vi "NMRvmeCard1.vi"() -> ()   [LabVIEW 2013]
uses:
  <vilib>/Utility/file.llb/Read From Spreadsheet File (DBL).vi
  <vilib>/Analysis/NI_AALBase.lvlib
panel:
  out "Telnet error out":errorcluster
  in  "Real/quad Q curve":bool=TRUE
  out "Temperature (C)":dbl(graph)=24.12
  out "+3V supply":dbl=3.245 format="%_4g"
  out "Temp (C)":dbl=24.12 format="%_4g"
  in  "RemovePed":bool=TRUE
  in  "IF / LOG Det":bool=TRUE
  in  "Q curve file":string="realback213.txt"
  out "File name 2":string="C:\\users\\plm\\Desktop\\rssmt\\realback213.txt"
  in  "AutoBaseline":bool
  out "RF OK":bool=TRUE
  out "Peak area (V-MHz)":sgl=0.0012676906 format="%.5f"
  in  "Gauss Fit":bool=TRUE
  out "NMR Graph + Fit":cluster{cluster{dbl, "Numeric":dbl}[]}[](graph)=[{[{224.37, "Numeric"=0.019981380952380993}, {224.372, "Numeric"=0.01883813333333495}, {224.374, "Numeric"=0.016386885714283997}, {224.376, "Numeric"=0.008227638095238155}, {224.37800000000001, "Numeric"=0.00466039047619202}, {224.38, "Numeric"=0.006385142857141357}, {224.382, "Numeric"=0.0035018952380952402}, {224.38400000000001, "Numeric"=0.005910647619049087}, {224.386, "Numeric"=0.004711399999998608}, {224.388, "Numeric"=0.005604152380952493}, {224.39000000000001, "Numeric"=0.0029889047619062}, {224.392, "Numeric"=0.006765657142855813}, {224.394, "Numeric"=0.00683440952380954}, {224.39600000000002, "Numeric"=0.006795161904763159}, {224.398, "Numeric"=0.002147914285713117}, {224.4, "Numeric"=0.002992666666666621}, {224.40200000000002, "Numeric"=-0.0024705809523797445}, {224.404, "Numeric"=0.00015817142857038526}, {224.406, "Numeric"=0.0007789238095238871}, {224.40800000000002, "Numeric"=-0.0025083238095228557}, {224.41, "Numeric"=-0.012503571428572361}, {224.412, "Numeric"=-0.009706819047619015}, {224.41400000000002, "Numeric"=-0.018818066666665807}, {224.416, "Numeric"=-0.01873731428571512}, {224.418, "Numeric"=-0.019264561904761987}, {224.42000000000002, "Numeric"=-0.012999809523808725}, {224.422, "Numeric"=-0.009943057142857946}, {224.424, "Numeric"=-0.00489430476190479}, {224.426, "Numeric"=-0.00615355238095111}, {224.428, "Numeric"=-0.0050208000000006485}, {224.43, "Numeric"=0.006503952380952323}, {224.432, "Numeric"=-0.003579295238094162}, {224.434, "Numeric"=-0.0057705428571434726}, {224.436, "Numeric"=-0.008969790476190571}, {224.438, "Numeric"=-0.009677038095237117}, {224.44, "Numeric"=-0.005792285714286235}, {224.442, "Numeric"=-0.004715533333333498}, {224.444, "Numeric"=-0.016146780952380223}, {224.446, "Numeric"=-0.01998602857142907}, {224.448, "Numeric"=-0.013633276190476386}, {224.45, "Numeric"=-0.009988523809523243}, {224.452, "Numeric"=0.002948228571428255}, {224.454, "Numeric"=0.009376980952380683}, {224.456, "Numeric"=0.013697733333333725}, {224.458, "Numeric"=0.01901048571428548}, {224.46, "Numeric"=0.030415238095237777}, {224.462, "Numeric"=0.037711990476190685}, {224.464, "Numeric"=0.0454007428571426}, {224.466, "Numeric"=0.060881495238094864}, {224.468, "Numeric"=0.07065424761904769}, {224.47, "Numeric"=0.07911899999999972}, {224.472, "Numeric"=0.07487575238095191}, {224.474, "Numeric"=0.06432450476190474}, {224.476, "Numeric"=0.055565257142856955}, {224.478, "Numeric"=0.03969800952380907}, {224.48, "Numeric"=0.019822761904761673}, {224.482, "Numeric"=0.012039514285714098}, {224.484, "Numeric"=0.0025482666666661463}, {224.486, "Numeric"=-0.004650980952381451}, {224.488, "Numeric"=-0.008758228571428682}, {224.49, "Numeric"=-0.009773476190476815}, {224.492, "Numeric"=-0.0021967238095244018}, {224.494, "Numeric"=-0.001127971428571451}, {224.496, "Numeric"=-0.0037672190476198773}, {224.498, "Numeric"=-0.0021144666666660606}, {224.5, "Numeric"=0.00043028571428570164}, {224.502, "Numeric"=-0.0007329619047626916}, {224.504, "Numeric"=0.0017957904761913349}, {224.506, "Numeric"=0.004616542857142707}, {224.508, "Numeric"=-0.00017070476190575782}, {224.51, "Numeric"=-0.001065952380951492}, {224.512, "Numeric"=-0.0026691999999999922}, {224.514, "Numeric"=-0.00778044761904867}, {224.516, "Numeric"=-0.0050996952380941585}, {224.518, "Numeric"=-0.005226942857142848}, {224.51999999999998, "Numeric"=-0.002862190476190984}, {224.522, "Numeric"=-0.004705438095236949}, {224.524, "Numeric"=-0.004856685714285773}, {224.52599999999998, "Numeric"=0.0025840666666660603}, {224.528, "Numeric"=0.009216819047620357}, {224.53, "Numeric"=0.0054415714285713495}, {224.53199999999998, "Numeric"=0.0009583238095230262}, {224.534, "Numeric"=-0.00043292380952248636}, {224.536, "Numeric"=0.0008678285714284759}, {224.53799999999998, "Numeric"=0.004360580952380025}, {224.54, "Numeric"=0.005645333333334857}, {224.542, "Numeric"=0.008922085714285575}, {224.54399999999998, "Numeric"=0.004790838095237049}, {224.546, "Numeric"=0.00255159047619202}, {224.548, "Numeric"=-0.009795657142857232}, {224.54999999999998, "Numeric"=-0.005650904761906031}, {224.552, "Numeric"=-0.0035141523809506803}, {224.554, "Numeric"=-0.004185400000000136}, {224.55599999999998, "Numeric"=-0.009264647619048945}, {224.558, "Numeric"=-0.0021518952380935015}, {224.56, "Numeric"=0.004852857142857059}, {224.56199999999998, "Numeric"=0.005449609523808043}, {224.564, "Numeric"=0.002138361904763719}, {224.566, "Numeric"=0.003119114285714139}, {224.56799999999998, "Numeric"=0.003891866666664966}, {224.57, "Numeric"=0.0027566190476209307}]}, {[{224.37, "Numeric"=4.996479157121043e-53}, {224.372, "Numeric"=5.331405671308769e-51}, {224.374, "Numeric"=5.17637625627724e-49}, {224.376, "Numeric"=4.573160046621097e-47}, {224.37800000000001, "Numeric"=3.6763209752488545e-45}, {224.38, "Numeric"=2.6891615986254814e-43}, {224.382, "Numeric"=1.7898920413809642e-41}, {224.38400000000001, "Numeric"=1.0840348153164538e-39}, {224.386, "Numeric"=5.974011869109323e-38}, {224.388, "Numeric"=2.9956797876429715e-36}, {224.39000000000001, "Numeric"=1.3668824093475549e-34}, {224.392, "Numeric"=5.675098152549435e-33}, {224.394, "Numeric"=2.143986553114384e-31}, {224.39600000000002, "Numeric"=7.370164723645891e-30}, {224.398, "Numeric"=2.3053601888071056e-28}, {224.4, "Numeric"=6.561556019740437e-27}, {224.40200000000002, "Numeric"=1.6993441869680083e-25}, {224.404, "Numeric"=4.004629265065266e-24}, {224.406, "Numeric"=8.587163671653244e-23}, {224.40800000000002, "Numeric"=1.6754968737140568e-21}, {224.41, "Numeric"=2.97470538953919e-20}, {224.412, "Numeric"=4.805634713914891e-19}, {224.41400000000002, "Numeric"=7.064216637569256e-18}, {224.416, "Numeric"=9.44895367190872e-17}, {224.418, "Numeric"=1.1500319007026123e-15}, {224.42000000000002, "Numeric"=1.2736277485103554e-14}, {224.422, "Numeric"=1.2834578034111644e-13}, {224.424, "Numeric"=1.1768663207807158e-12}, {224.426, "Numeric"=9.819268406815462e-12}, {224.428, "Numeric"=7.45482728048275e-11}, {224.43, "Numeric"=5.149943891555167e-10}, {224.432, "Numeric"=3.2372323103657745e-09}, {224.434, "Numeric"=1.851619273182036e-08}, {224.436, "Numeric"=9.636869461784531e-08}, {224.438, "Numeric"=4.5638011879864213e-07}, {224.44, "Numeric"=1.966635685025587e-06}, {224.442, "Numeric"=7.711299494825998e-06}, {224.444, "Numeric"=2.7512983238559256e-05}, {224.446, "Numeric"=8.932113926203351e-05}, {224.448, "Numeric"=0.0002638622619953867}, {224.45, "Numeric"=0.0007092621201427087}, {224.452, "Numeric"=0.0017347732149989375}, {224.454, "Numeric"=0.0038608693662806003}, {224.456, "Numeric"=0.007818689455772231}, {224.458, "Numeric"=0.014407521558145594}, {224.46, "Numeric"=0.024157447780126944}, {224.462, "Numeric"=0.03685694020534238}, {224.464, "Numeric"=0.05116747240443425}, {224.466, "Numeric"=0.06463609450757957}, {224.468, "Numeric"=0.0742955338825832}, {224.47, "Numeric"=0.07770639578127585}, {224.472, "Numeric"=0.0739532527937006}, {224.474, "Numeric"=0.0640419066890079}, {224.476, "Numeric"=0.050463536567084744}, {224.478, "Numeric"=0.036182416660317206}, {224.48, "Numeric"=0.02360608219203614}, {224.482, "Numeric"=0.014013825865809171}, {224.484, "Numeric"=0.007570001678288115}, {224.486, "Numeric"=0.0037208459705686692}, {224.488, "Numeric"=0.0016641553514492678}, {224.49, "Numeric"=0.0006772554318493228}, {224.492, "Numeric"=0.0002507942558558377}, {224.494, "Numeric"=8.450630852905024e-05}, {224.496, "Numeric"=2.59099833493484e-05}, {224.498, "Numeric"=7.228556737491606e-06}, {224.5, "Numeric"=1.8350272242305546e-06}, {224.502, "Numeric"=4.2387703390211724e-07}, {224.504, "Numeric"=8.90930278726135e-08}, {224.506, "Numeric"=1.7039388635256535e-08}, {224.508, "Numeric"=2.965314459410487e-09}, {224.51, "Numeric"=4.69563098204409e-10}, {224.512, "Numeric"=6.765869563309472e-11}, {224.514, "Numeric"=8.870737740659163e-12}, {224.516, "Numeric"=1.0582842087595977e-12}, {224.518, "Numeric"=1.1488183111935901e-13}, {224.51999999999998, "Numeric"=1.1347673718942467e-14}, {224.522, "Numeric"=1.0199262936518405e-15}, {224.524, "Numeric"=8.341366305650706e-17}, {224.52599999999998, "Numeric"=6.20743321960535e-18}, {224.528, "Numeric"=4.2033289216604396e-19}, {224.53, "Numeric"=2.5898890134957684e-20}, {224.53199999999998, "Numeric"=1.4520293268026514e-21}, {224.534, "Numeric"=7.407575384802874e-23}, {224.536, "Numeric"=3.4386124328008906e-24}, {224.53799999999998, "Numeric"=1.4524354344352625e-25}, {224.54, "Numeric"=5.582347908555169e-27}, {224.542, "Numeric"=1.9522859135246242e-28}, {224.54399999999998, "Numeric"=6.2126430133960394e-30}, {224.546, "Numeric"=1.7989365057346025e-31}, {224.548, "Numeric"=4.7398186788252815e-33}, {224.54999999999998, "Numeric"=1.1363551343839747e-34}, {224.552, "Numeric"=2.478979219883001e-36}, {224.554, "Numeric"=4.920827616420029e-38}, {224.55599999999998, "Numeric"=8.888119269018469e-40}, {224.558, "Numeric"=1.4607908954776238e-41}, {224.56, "Numeric"=2.1846038284560563e-43}, {224.56199999999998, "Numeric"=2.9727869424363234e-45}, {224.564, "Numeric"=3.6809620192977223e-47}, {224.566, "Numeric"=4.147298983609085e-49}, {224.56799999999998, "Numeric"=4.2518292134929295e-51}, {224.57, "Numeric"=3.966365529511812e-53}]}]
  in  "Amp of Q curve":dbl=0.9999999999999999 min=0.0 max=7.0 step=0.01 format="%_3f"
  in  "Subtract Q curve":bool=TRUE
  in  "Adjust Tune":bool
  out "Pedestal Offset":dbl(graph)=0.7186800000000002
  out "Pedestal Difference":dbl(graph)=0.003027333333333382
  out "# Good Spectra":i32=97
  in  "Quality cuts":bool=TRUE
  out "Pedestal OK":bool=TRUE
  out "Sweep #":i32=127
  out "1st Sweep":bool
  out "ADC volts OK":bool=TRUE
  out "Peak Height Distribution":cluster{"Y":dbl[], "Y":dbl[]}[](graph)=[{"Y"=[0.04386130127363737, 0.04436487009623908, 0.0448684389188408, 0.04537200774144251, 0.04587557656404422, 0.04637914538664594, 0.04688271420924765, 0.04738628303184937, 0.04788985185445108, 0.048393420677052795, 0.048896989499654514, 0.049400558322256226, 0.049904127144857945, 0.050407695967459656, 0.050911264790061375, 0.05141483361266309, 0.0519184024352648, 0.05242197125786652, 0.05292554008046823, 0.05342910890306995, 0.05393267772567166, 0.05443624654827338, 0.05493981537087509, 0.0554433841934768, 0.05594695301607852, 0.05645052183868023, 0.05695409066128195, 0.057457659483883664, 0.057961228306485375, 0.058464797129087094, 0.058968365951688806, 0.059471934774290525, 0.059975503596892236, 0.060479072419493955, 0.06098264124209567, 0.06148621006469738, 0.0619897788872991, 0.06249334770990081, 0.06299691653250253, 0.06350048535510425, 0.06400405417770595, 0.06450762300030767, 0.06501119182290939, 0.0655147606455111, 0.06601832946811281, 0.06652189829071453, 0.06702546711331625, 0.06752903593591796, 0.06803260475851967, 0.06853617358112139, 0.0690397424037231, 0.06954331122632482, 0.07004688004892654, 0.07055044887152824, 0.07105401769412996, 0.07155758651673168, 0.0720611553393334, 0.0725647241619351, 0.07306829298453682, 0.07357186180713854, 0.07407543062974024, 0.07457899945234196, 0.07508256827494368, 0.0755861370975454, 0.0760897059201471, 0.07659327474274882, 0.07709684356535054, 0.07760041238795225, 0.07810398121055397, 0.07860755003315568, 0.0791111188557574, 0.07961468767835911, 0.08011825650096083, 0.08062182532356255, 0.08112539414616425, 0.08162896296876597, 0.08213253179136769, 0.08263610061396941, 0.08313966943657111, 0.08364323825917283, 0.08414680708177455, 0.08465037590437625, 0.08515394472697797, 0.08565751354957969, 0.0861610823721814, 0.08666465119478312, 0.08716822001738483, 0.08767178883998655, 0.08817535766258826, 0.08867892648518998, 0.0891824953077917, 0.0896860641303934, 0.09018963295299512, 0.09069320177559684, 0.09119677059819856, 0.09170033942080026, 0.09220390824340198, 0.0927074770660037, 0.0932110458886054, 0.09371461471120712], "Y"=[1.0, 0.0, 0.0, 0.0, 0.0, 0.0, 2.0, 0.0, 0.0, 0.0, 0.0, 0.0, 0.0, 0.0, 0.0, 0.0, 0.0, 0.0, 0.0, 0.0, 0.0, 0.0, 2.0, 1.0, 0.0, 0.0, 0.0, 0.0, 1.0, 0.0, 0.0, 3.0, 0.0, 2.0, 0.0, 1.0, 0.0, 1.0, 1.0, 0.0, 0.0, 0.0, 2.0, 2.0, 1.0, 1.0, 1.0, 2.0, 1.0, 0.0, 6.0, 1.0, 1.0, 1.0, 2.0, 2.0, 5.0, 0.0, 3.0, 3.0, 4.0, 1.0, 2.0, 0.0, 3.0, 2.0, 1.0, 2.0, 3.0, 2.0, 0.0, 3.0, 1.0, 0.0, 0.0, 1.0, 2.0, 2.0, 1.0, 1.0, 1.0, 2.0, 0.0, 1.0, 1.0, 2.0, 0.0, 3.0, 1.0, 1.0, 0.0, 1.0, 0.0, 0.0, 2.0, 0.0, 0.0, 0.0, 1.0, 1.0]}]
  in  "# of Sweeps":i32=1000
  out "S/N":dbl=7.101836430067523 format="%_3g"
  out "Peak mean (V)":dbl=0.07363174247132291 format="%_4g"
  out "Peak Height":dbl(graph)=0.0777085900348737
  in  "Raw Data":bool=TRUE
  in  "Tank RF":bool=TRUE
  in  "IF Atten (dB)":i8=9 min=0 max=31 step=1
  in  "IFoffset (V)":dbl=6.713 min=-0.0 max=8.0 step=0.001 format="%.4f"
  in  "Tune  (V)":dbl=2.6299999999999994 min=0.0 max=5.0 step=0.001 format="%.4f"
  in  "Hi / Lo IF Gain":bool
  out "Voltage Array":sgl[](array[numeric])=[0.7467, 0.7452, 0.7424, 0.7339, 0.73, 0.7314, 0.7282, 0.7303, 0.7288, 0.7294, 0.7265, 0.73, 0.7298, 0.7295, 0.7246, 0.7252, 0.7195, 0.7219, 0.7223, 0.7188, 0.7086, 0.7112, 0.7019, 0.7018, 0.7011, 0.7072, 0.7101, 0.715, 0.7136, 0.7146, 0.726, 0.7158, 0.7135, 0.7102, 0.7094, 0.7132, 0.7142, 0.7027, 0.6988, 0.7051, 0.7087, 0.7216, 0.728, 0.7323, 0.7376, 0.749, 0.7563, 0.764, 0.7795, 0.7893, 0.7978, 0.7936, 0.7831, 0.7744, 0.7586, 0.7388, 0.7311, 0.7217, 0.7146, 0.7106, 0.7097, 0.7174, 0.7186, 0.7161, 0.7179, 0.7206, 0.7196, 0.7223, 0.7253, 0.7207, 0.72, 0.7186, 0.7137, 0.7166, 0.7167, 0.7193, 0.7177, 0.7178, 0.7255, 0.7324, 0.7289, 0.7247, 0.7236, 0.7252, 0.729, 0.7306, 0.7342, 0.7304, 0.7285, 0.7165, 0.721, 0.7235, 0.7232, 0.7185, 0.726, 0.7334, 0.7344, 0.7315, 0.7329, 0.7341, 0.7334] format="%.4f"
  in  "Invert Polarity":bool
  out "Pedestal Diff (V)":sgl=0.0030273334 format="%.3f"
  out "Peak amp (V)":sgl=0.07770859 format="%.3f"
  in  "Save Data to File":bool
  in  "RF Level (dBm)":dbl min=-10.0 max=10.0 step=0.1 format="%.2f"
  out "SMT error out":errorcluster
  out "Sample RMS (V)":dbl=0.001420792079207921 format="%.4f"
  in  "# Sample/step":i32=100 min=1 max=1000 step=100
  in  "Step Width (MHz)":dbl=0.002 min=0.0 max=1000.0 step=0.0005 format="%.4f"
  in  "Freq Span (MHz)":dbl=0.2 min=0.0 max=3000.0 step=0.1 format="%.3f"
  in  "Center Freq (MHz)":dbl=224.47 min=0.005 max=6000.0 step=0.1 format="%.3f"
  in  "Sweep Mode":u16(ring)=3 items=["Off", "Single", "Auto", "Step"]
  in  "GPIB Addr (28)":refnum<visa-resource-name>="GPIB0::28::INSTR"
  # "E1039 Prototype NMR Control Panel"
  # "Settings"
  # "D\nA\nC"
  # "R\nF\n\nG\nE\nN \n\n+\n\nI\nF"
  # "A\nD\nC"
  # "D\nA\nT\nA\n\n+\n\nA \nN\nA\nL\nY\nS\nI\nS"
  # "I\n/\nO"
  # "Results"
  # "A\nv\ne\nr\na\ng\ne"
  # "S\nw\ne\ne\np"
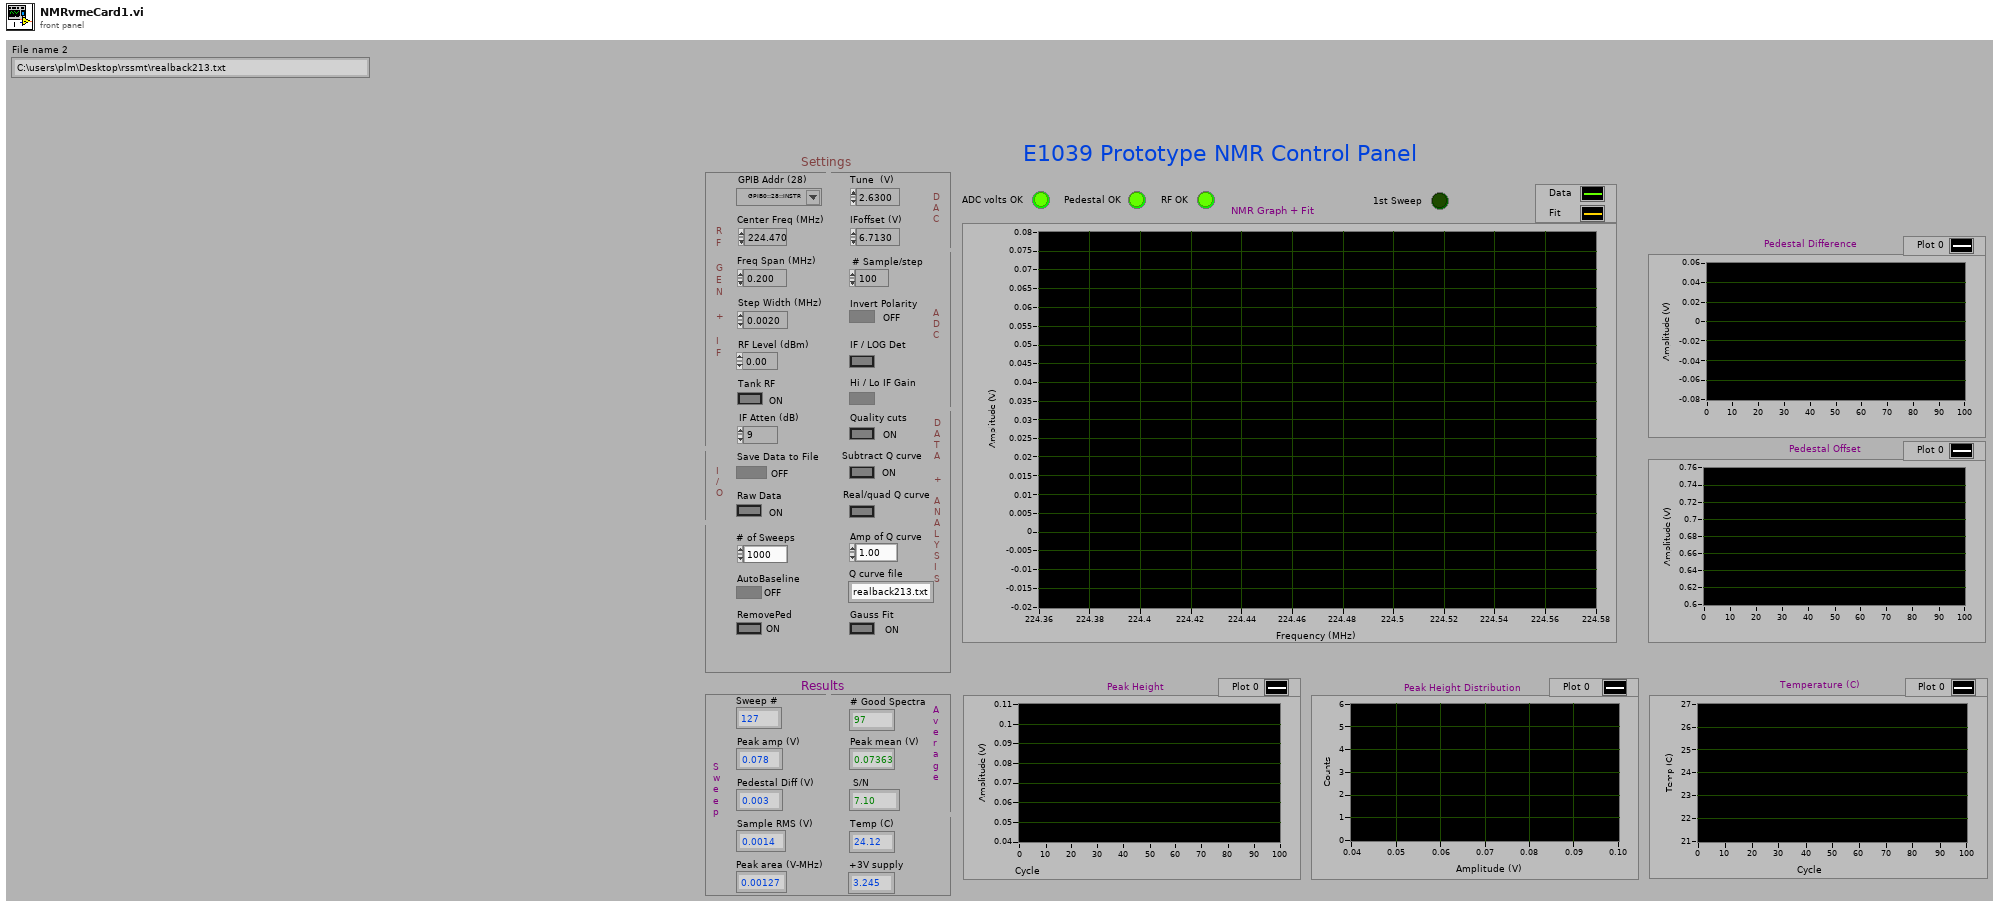
[diagram p1: front panel]
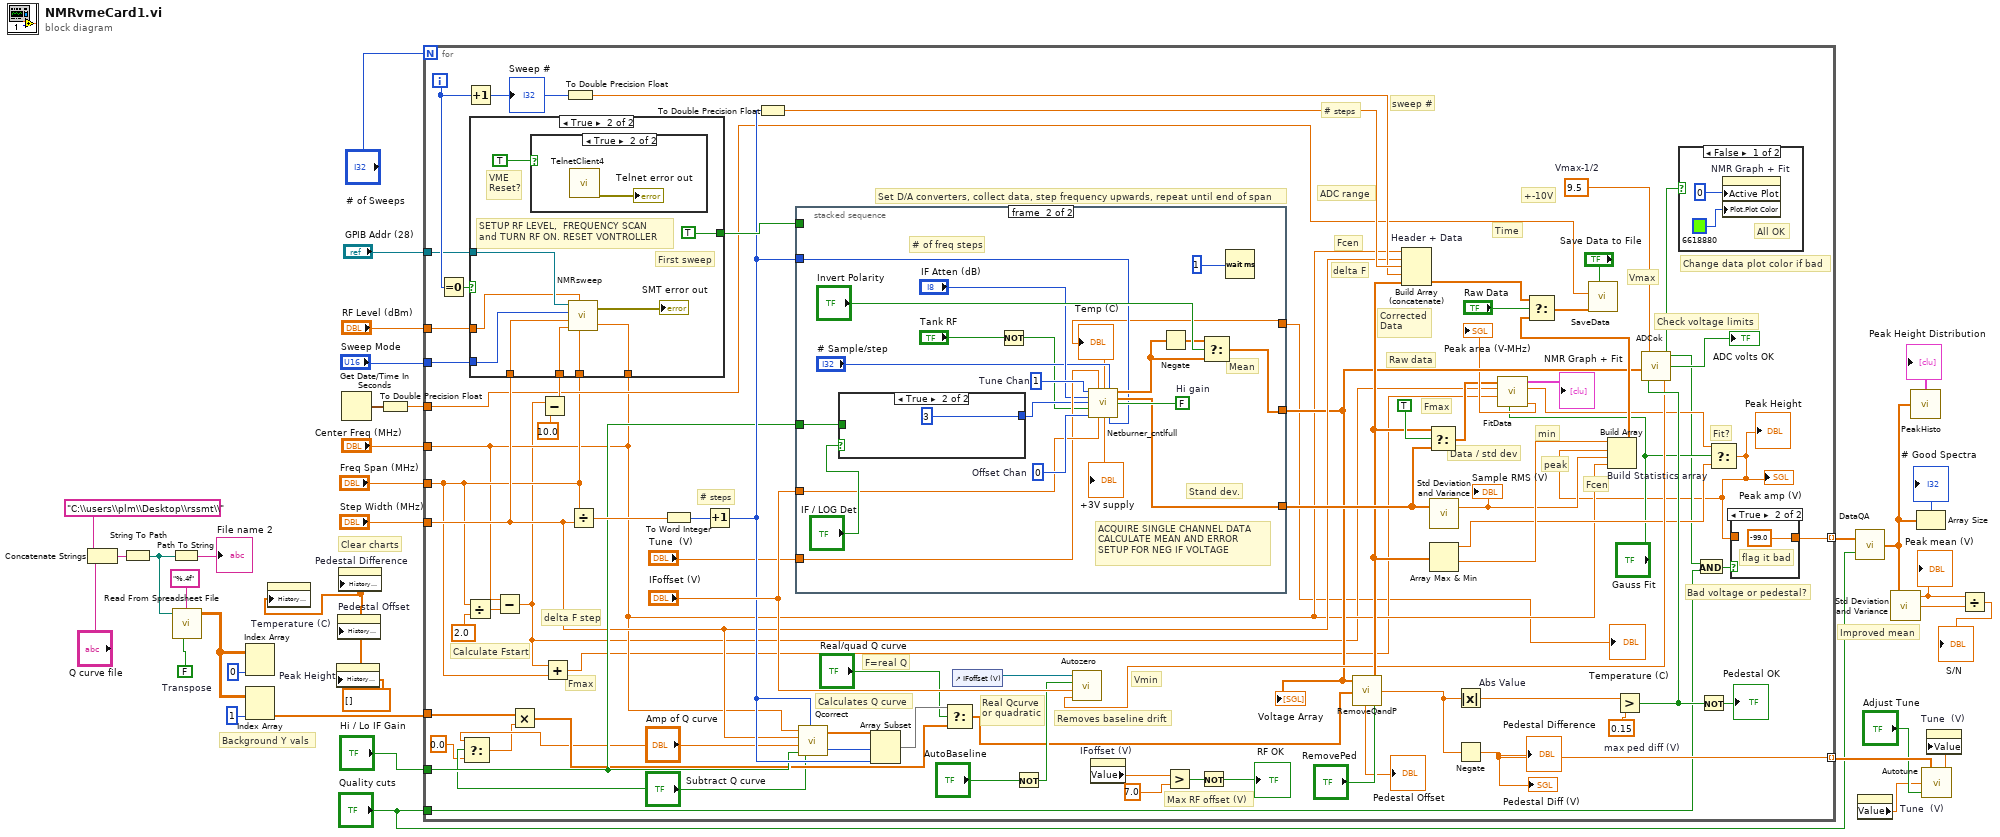
[diagram p0: block diagram]
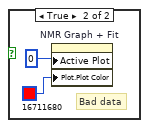
[diagram p2: hidden frame]
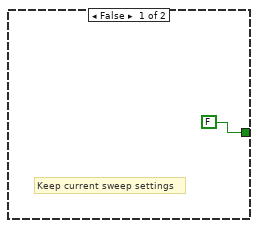
[diagram p4: hidden frame]
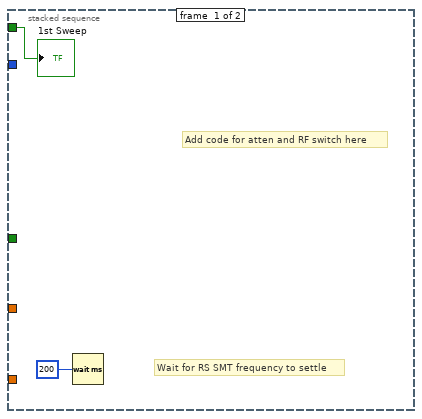
[diagram p6: hidden frame]
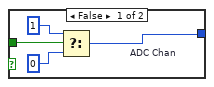
[diagram p7: hidden frame]
diagram:
  w12 = FALSE  # Transpose
  w4 = dbl[] []
  # "Background Y vals"
  # "Clear charts"
  # "Improved mean"
  n1 = Concatenate Strings "Concatenate Strings"("C:\\users\\plm\\Desktop\\rssmt\\", "Q curve file") -> (w15:string)
  n2 = String To Path(string=w15) -> (path=w11:path)
  n3 = Path To String(path=w11) -> (string=→"File name 2":string)
  n4 = call-poly <vilib>:"Read From Spreadsheet File.vi"("transpose (no:F)"=w12, "format (%.3f)"="%.4f", "file path (dialog if empty)"=w11) -> ("all rows"=w10:dbl[][])  [unwired: 4 in, 4 out]
  n5 = Index Array "Index Array"(array=w10, index (col)=0) -> ()  [unwired: 1 in, 1 out]
  n6 = Index Array(array=w10, index (col)=1) -> (element=w5:dbl[])  [unwired: 1 in]
  n7 = property on="Temperature (C)" class="WFChart (strict)"("History Data"=w4) -> ()  [unwired: 2 in, 2 out]
  n8 = property on="Peak Height" class="WFChart (strict)"("History Data"=w4) -> ()  [unwired: 2 in, 2 out]
  n9 = property on="Pedestal Offset" class="WFChart (strict)"("History Data"=w4) -> ()  [unwired: 2 in, 2 out]
  n10 = property on="Pedestal Difference" class="WFChart (strict)"("History Data"=w4) -> ()  [unwired: 2 in, 2 out]
  n11 = Get Date/Time In Seconds() -> (seconds since 1Jan1904=w17:timestamp)
  n12 = To Double Precision Float(number=w17) -> (double precision float=w16:dbl)
  n13 = for {
    N: "# of Sweeps" -> [_]
    tunnel: [w95] -> w32 mode=indexing
    tunnel: "Quality cuts" -> [w72]
    tunnel: [w78] -> w29 mode=indexing
    tunnel: "Center Freq (MHz)" -> [w59]
    tunnel: "Freq Span (MHz)" -> [w65]
    tunnel: "Step Width (MHz)" -> [w71]
    tunnel: "Sweep Mode" -> [w82]
    tunnel: "Hi / Lo IF Gain" -> [w81]
    tunnel: "GPIB Addr (28)" -> [w80]
    tunnel: "RF Level (dBm)" -> [w79]
    tunnel: w16 -> [w66]
    tunnel: w5 -> [w44]
    i -> [w93]
    w76 = 9.5  # Vmax-1/2
    w96 = 0.15  # max ped diff (V)
    # "F=real Q"
    # "Real Qcurve\nor quadratic"
    # "+-10V"
    # "Vmax"
    # "Change data plot color if bad"
    # "Max RF offset (V)"
    # "Fmax"
    # "Fit?"
    # "Fmax"
    # "Time"
    # "Vmin"
    # "min"
    # "peak"
    # "Raw data"
    # "Corrected\nData"
    # "Fcen"
    # "delta F"
    # "# steps"
    # "ADC range"
    # "sweep #"
    # "Fcen"
    # "Set D/A converters, collect data, step frequency upwards, repeat until end of span"
    # "Calculates Q curve"
    # "Removes baseline drift"
    # "Bad voltage or pedestal?"
    # "Check voltage limits"
    # "Data / std dev"
    # "# steps"
    # "Calculate Fstart"
    # "delta F step"
    n14 = Equal To 0?(x=w93) -> (x = 0?=w98:bool)
    n15 = Select(t="Amp of Q curve", s="Subtract Q curve", f=0.0) -> (s? t:f=w39:dbl)
    n16 = Divide(x=w65, y=sgl 2.0) -> (x/y=w109:dbl)
    n17 = Increment(x=w93) -> (x+1=w83:i32)
    "Sweep #" <- w83
    n18 = Subtract(x=w59, y=w109) -> (x-y=w54:dbl)
    n19 = Multiply(x=w44, y=w39) -> (x*y=w43:dbl[])
    n20 = Subtract(x=w54, y=10.0) -> (x-y=w107:dbl)
    n21 = case shown="True" w98 {
      tunnel: w107 -> [_ w128]
      tunnel: w71 -> [_ w126]
      tunnel: w59 -> [_ w125]
      tunnel: w65 -> [_ w127]
      tunnel: [FALSE TRUE] -> w97
      tunnel: w82 -> [_ w122]
      tunnel: w80 -> [_ w121]
      tunnel: w79 -> [_ w120]
      frame False {
        # "Keep current sweep settings"
      }
      frame True {
        # "VME\nReset?"
        # "First sweep"
        # "SETUP RF LEVEL,  FREQUENCY SCAN\nand TURN RF ON. RESET VONTROLLER"
        n22 = case shown="True" TRUE {
          frame False {
          }
          frame True {
            n23 = call "TelnetClient4.vi"() -> ("Telnet error"=→"Telnet error out":errorcluster)  [unwired: 4 in, 3 out]
          }
        }
        n24 = call "NMRsweep.vi"("Center Freq (MHz)"=w125, "Freq Span (MHz)"=w127, "RF Level (dBm)"=w120, "Foffset (MHz)"=w128, "Step Width (MHz)"=w126, "Sweep Mode"=w122, "GPIB Addr (28)"=w121) -> ("error out"=→"SMT error out":errorcluster)
      }
    }
    n25 = Add(x=w54, y=w65) -> (x+y=w53:dbl)
    n26 = To Double Precision Float(number=w83) -> (double precision float=w84:dbl)
    n27 = Divide(x=w65, y=w71) -> (x/y=w111:dbl)
    n28 = To Word Integer(number=w111) -> (16bit integer=w108:i16)
    n29 = Increment(x=w108) -> (x+1=w87:i16)
    n30 = To Double Precision Float(number=w87) -> (double precision float=w86:dbl)
    n31 = stacked-sequence {
      tunnel: [_ w139] -> w101
      tunnel: [_ w150] -> w69
      tunnel: w87 -> [_ w136]
      tunnel: "IFoffset (V)" -> [_ w145]
      tunnel: w81 -> [_ w148]
      tunnel: w97 -> [w130 _]
      tunnel: "Tune  (V)" -> [_ w143]
      tunnel: [_ w134] -> w35
      frame #0 {
        # "Add code for atten and RF switch here"
        # "Wait for RS SMT frequency to settle"
        n32 = Wait (ms)(milliseconds to wait=200) -> ()  [unwired: 1 out]
        "1st Sweep" <- w130
      }
      frame #1 {
        w141 = FALSE  # Hi gain
        w146 = 0  # Offset Chan
        w144 = 1  # Tune Chan
        # "Stand dev."
        # "Mean"
        # "ACQUIRE SINGLE CHANNEL DATA\nCALCULATE MEAN AND ERROR\nSETUP FOR NEG IF VOLTAGE"
        # "# of freq steps"
        n33 = case shown="True" "IF / LOG Det" {
          tunnel: w148 -> [w156 _]
          tunnel: [w153 3] -> w138
          frame False {
            n34 = Select "ADC Chan"(t=1, s=w156, f=0) -> (s? t:f=w153:i32)
          }
          frame True {
          }
        }
        n35 = Not(x="Tank RF") -> (.not. x?=w133:bool)
        n36 = call "Netburner_cntlfull.vi"("Tune DAC"=w144, "Tune Volt"=w143, "# Data"="# Sample/step", "IF Atten (dB)"="IF Atten (dB)", "NMR ADC"=w138, "Hi Gain"=w141, "Tank RF"=w133, "Offset DAC"=w146, "Offset Volt"=w145, "# f steps"=w136) -> ("Temp (C)"=w134:dbl, "ADC value"=w140:dbl[], "ADC error"=w139:dbl[], "Volts"=→"+3V supply":dbl)  [unwired: 2 out]
        "Temp (C)" <- w134
        n37 = Negate(x=w140) -> (-x=w149:dbl[])
        n38 = Select(t=w149, s="Invert Polarity", f=w140) -> (s? t:f=w150:dbl[])
        n39 = Wait (ms)(milliseconds to wait=1) -> ()  [unwired: 1 out]
      }
    }
    "Voltage Array" <- w69
    "Temperature (C)" <- w35
    n40 = call "Qcorrect.vi"("Subtract Q curve"="Subtract Q curve", "Nstep"=w87, "IF or Log"=w81, "Amp of Q curve"="Amp of Q curve", "Step Width (MHz)"=w71, "Center Freq (MHz)"=w59) -> ("Start"=w102:i32, "Array"=w103:dbl[])
    n41 = Array Subset "Array Subset"(array=w103, index=w102, length=w87) -> (w47:dbl[])
    n42 = Select(t=w47, s="Real/quad Q curve", f=w43) -> (s? t:f=w46:dbl[])
    n43 = control-ref of="IFoffset (V)"() -> (w75:refnum<vi>)
    n44 = Not(x="AutoBaseline") -> (.not. x?=w48:bool)
    n45 = property on="IFoffset (V)" class="DigNum (strict)"() -> ("Value"=w63:dbl)  [unwired: 2 in, 2 out]
    n46 = Greater?(x=w63, y=7.0) -> (0:w61:bool)
    n47 = Not(x=w61) -> (.not. x?=→"RF OK":bool)
    n48 = call "RemoveQandP.vi"("Subtract Ped?"="RemovePed", "Qcurve"=w46, "Raw data"=w69) -> ("Ped L-R"=w89:dbl, "Corrected data"=w85:dbl[], "Ped Offfset"=→"Pedestal Offset":dbl)
    n49 = Build Array (concatenate) "Header + Data"(w59, w71, w86, w84, w85) -> (w88:dbl[])
    n50 = Select(t=w85, s=TRUE, f=w101) -> (s? t:f=w55:dbl[])
    n51 = call <vilib>:"Std Deviation and Variance.vi"("X"=w101) -> ("mean"=w70:dbl)  [unwired: 1 in, 2 out]
    "Sample RMS (V)" <- w70
    n52 = Array Max & Min(array=w85) -> (max value=w64:dbl, min value=w100:dbl)  [unwired: 2 out]
    n53 = Absolute Value "Abs Value"(x=w89) -> (abs(x)=w91:dbl)
    n54 = Negate(x=w89) -> (-x=w78:dbl)
    "Pedestal Diff (V)" <- w78
    "Pedestal Difference" <- w78
    n55 = call "FitData.vi"("Fit?"="Gauss Fit", "Fmax"=w53, "Fmin"=w54, "Yarray"=w55) -> ("Peak Area (V-MHz)"=→"Peak area (V-MHz)":dbl, "Amplitude (V)"=w57:dbl, "NMR Graph + Fit"=→"NMR Graph + Fit":cluster{cluster{dbl, "Numeric":dbl}[]}[])  [unwired: 2 out]
    n56 = Greater?(x=w91, y=w96) -> (0:w77:bool)
    n57 = call "ADCok.vi"("PedOK"=w77, "Array"=w69, "Vmax-1/2"=w76) -> ("Vmin"=w74:dbl, "ADC voltages OK"=→"ADC volts OK":bool, "Allok"=w51:bool)
    n58 = call "Autozero.vi"("Vmin (V)"=w74, "IFoffset (V)"="IFoffset (V)", "IF or Log"=w48, "reference"=w75) -> ()
    n59 = case shown="False" w51 {
      frame False {
        # "All OK"
        n60 = property on="NMR Graph + Fit" class="XYGraph (strict)"("Active Plot"=0, "Plot.Plot Color"=u32 6618880) -> ()  [unwired: 2 in, 2 out]
      }
      frame True {
        # "Bad data"
        n61 = property on="NMR Graph + Fit" class="XYGraph (strict)"("Active Plot"=0, "Plot.Plot Color"=u32 16711680) -> ()  [unwired: 2 in, 2 out]
      }
    }
    n62 = And(x=w51, y=w72) -> (x .and. y?=w92:bool)
    n63 = Not(x=w77) -> (.not. x?=→"Pedestal OK":bool)
    n64 = Select(t=w57, s="Gauss Fit", f=w64) -> (s? t:f=w50:dbl)
    "Peak amp (V)" <- w50
    "Peak Height" <- w50
    n65 = Build Array "Build Statistics array"(w100, w50, w70, w59) -> (w106:dbl[])
    n66 = Select(t=w88, s="Raw Data", f=w106) -> (s? t:f=w67:dbl[])
    n67 = call "SaveData.vi"("Array"=w67, "Save Data to File"="Save Data to File", "Ext time (sec)"=w66) -> ()  [unwired: 1 out]
    n68 = case shown="True" w92 {
      tunnel: [w116 -99.0] -> w95
      tunnel: w50 -> [w116 _]
      frame False {
        # "Data OK"
      }
      frame True {
        # "flag it bad"
      }
    }
  }
  n69 = call "DataQA.vi"("Quality cuts"="Quality cuts", "Data In"=w32) -> ("Data Out"=w31:dbl[])
  n70 = property on="Tune  (V)" class="DigNum (strict)"() -> ("Value"=w20:dbl)  [unwired: 2 in, 2 out]
  n71 = call <vilib>:"Std Deviation and Variance.vi"("X"=w31) -> ("mean"=w3:dbl, "standard deviation"=w2:dbl)  [unwired: 1 in, 1 out]
  "Peak mean (V)" <- w3
  n72 = call "PeakHisto.vi"("Data Out"=w31) -> ("XY Graph"=→"Peak Height Distribution":cluster{"Y":dbl[], "Y":dbl[]}[])
  n73 = Array Size(array=w31) -> (size(s)=→"# Good Spectra":i32)
  n74 = call "Autotune.vi"("Adjust Tune"="Adjust Tune", "Tune Vin"=w20, "Pedestal Diff"=w29) -> ("Tune Vout"=w19:dbl)
  n75 = property on="Tune  (V)" class="DigNum (strict)"("Value"=w19) -> ()  [unwired: 2 in, 2 out]
  n76 = Divide(x=w3, y=w2) -> (x/y=→"S/N":dbl)
